vi "Compare Two Paths__ogtk.vi"   [LabVIEW 2014]
doc: "Compare Two Paths.vi - Compares two paths and if the paths are the same type (both absolute or both relative), the relative path between them is returned."
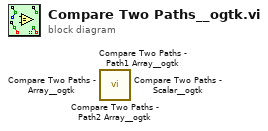
[diagram p0: block diagram]
diagram:
  n1 = call <userlib>:"Compare Two Paths - Path2 Array__ogtk.vi"() -> ()  [unwired: 3 in, 3 out]
  n2 = call <userlib>:"Compare Two Paths - Path1 Array__ogtk.vi"() -> ()  [unwired: 3 in, 3 out]
  n3 = call <userlib>:"Compare Two Paths - Array__ogtk.vi"() -> ()  [unwired: 3 in, 3 out]
  n4 = call <userlib>:"Compare Two Paths - Scalar__ogtk.vi"() -> ()  [unwired: 3 in, 3 out]
